vi "getViPath.vi"() -> (3 "VI Path":path)   [LabVIEW 2017, in "BuildWorker Controller.lvlib" / "BuildWorker Controller.lvclass"]
uses:
  BuildWorker Controller.lvclass
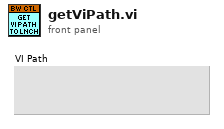
[diagram p1: front panel]
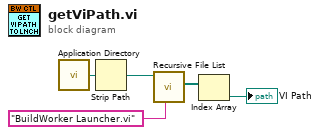
[diagram p0: block diagram]
diagram:
  n1 = call <vilib>:"Application Directory.vi"() -> ("Application Directory"=w4:path)
  n2 = Strip Path(path=w4) -> (stripped path=w1:path)  [unwired: 1 out]
  n3 = call <vilib>:"Recursive File List.vi"("pattern"="BuildWorker Launcher.vi" ("VI Path"), "Folder Path"=w1) -> ("All Files in Dir"=w3:path[])  [unwired: 5 in, 4 out]
  n4 = Index Array(array=w3) -> (element=→"VI Path":path)  [unwired: 1 in]
